vi "Shooter Teleop.vi"(11 "Cluster":T1={"Axes Right"=[], " Axes Left"=[], " Axes Co-driver"=[-0.015748031496062992, -0.015748031496062992, 0.0, 0.0, 0.03937007874015748, -0.031496062992125984], "Buttons Right"=[], "Buttons Left"=[], "Buttons Co-driver"=[FALSE, FALSE, FALSE, FALSE, FALSE, FALSE, FALSE, FALSE, FALSE, FALSE], "POVs Right"=[], "POVs Left"=[], "POVs Co-driver"=[-1]}) -> ()   [LabVIEW 2016]
uses:
  Joystick vals.ctl
  <vilib>/Rock Robotics/Network Tables/NT Read Number.vi
panel:
  in  "top POV":dbl=-90.0 format="%#_13g"
  in  "90":dbl format="%#_13g"
  in  "180":dbl=90.0 format="%#_13g"
  in  "Speed":dbl=3500.0 format="%#_13g"
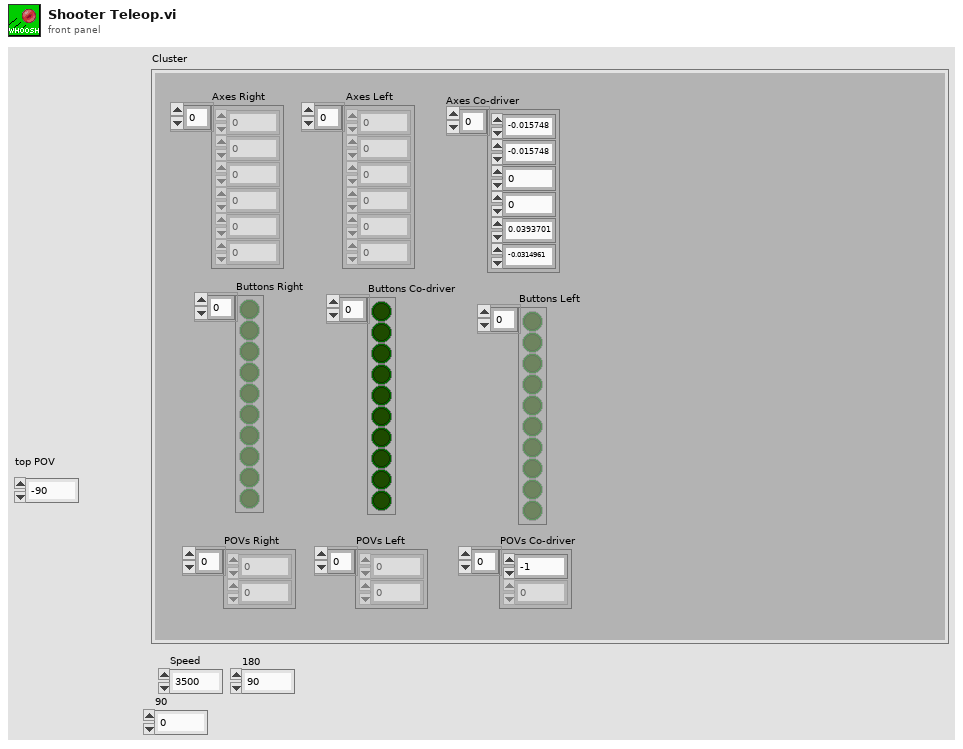
[diagram p1: front panel]
types:
  T1 = typedef "Joystick vals.ctl" = cluster{"Axes Right":dbl[], " Axes Left":dbl[], " Axes Co-driver":dbl[], "Buttons Right":bool[], "Buttons Left":bool[], "Buttons Co-driver":bool[], "POVs Right":i16[], "POVs Left":i16[], "POVs Co-driver":i16[]}
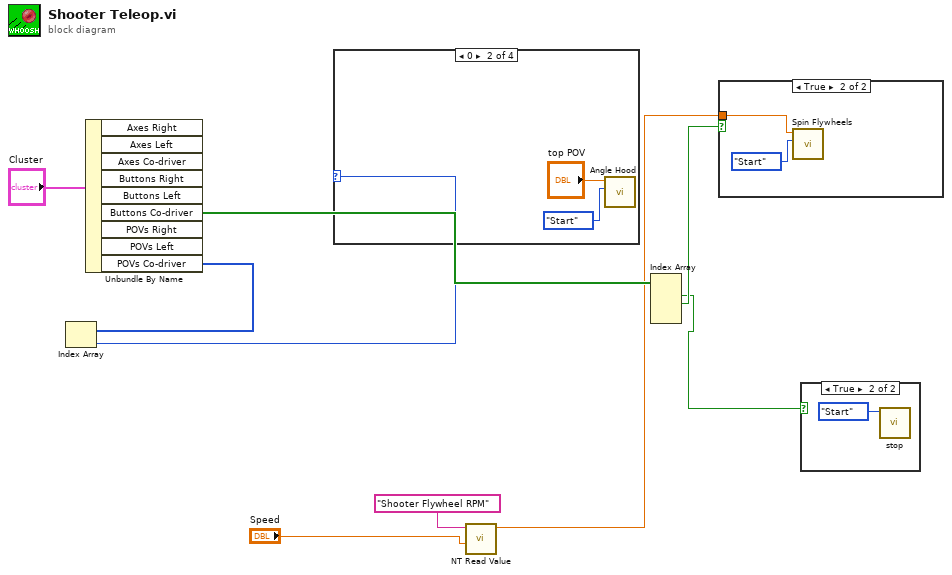
[diagram p0: block diagram]
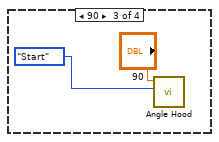
[diagram p3: hidden frame]
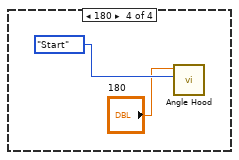
[diagram p4: hidden frame]
diagram:
  n1 = Unbundle By Name("Cluster") -> ("Buttons Co-driver"=w7:bool[], "POVs Co-driver"=w6:i16[])  [unwired: 7 out]
  n2 = Index Array(array=w6) -> (element=w5:i16)  [unwired: 1 in]
  n3 = case shown="0" w5 {
    frame -1, Default {
    }
    frame 0 {
      n4 = call "Angle Hood.vi"("Synchronication"=enum16{"Start", "Wait"}."Start", "Angle Hood"="top POV") -> ()  [unwired: 9 in, 1 out]
    }
    frame 90 {
      n5 = call "Angle Hood.vi"("Synchronication"=enum16{"Start", "Wait"}."Start", "Angle Hood"="90") -> ()  [unwired: 9 in, 1 out]
    }
    frame 180 {
      n6 = call "Angle Hood.vi"("Synchronication"=enum16{"Start", "Wait"}."Start", "Angle Hood"="180") -> ()  [unwired: 9 in, 1 out]
    }
  }
  n7 = call-poly <vilib>:"NT Read Value.vi"("Default Value"="Speed", "Name"="Shooter Flywheel RPM") -> ("Numeric"=w1:dbl)  [unwired: 8 in, 1 out]
  n8 = Index Array(array=w7) -> (element #1=w2:bool, element #2=w8:bool)  [unwired: 4 in, 2 out]
  n9 = case shown="True" w8 {
    tunnel: w1 -> [_ w16]
    frame False {
    }
    frame True {
      n10 = call "Spin Flywheels.vi"("Synchronication"=enum16{"Start", "Wait"}."Start", "Speed RPM"=w16) -> ()  [unwired: 9 in, 1 out]
    }
  }
  n11 = case shown="True" w2 {
    frame False {
    }
    frame True {
      n12 = call "stop.vi"("Synchronication"=enum16{"Start", "Wait"}."Start") -> ()  [unwired: 10 in, 1 out]
    }
  }
